vi "Create Custom Device.vi"(8 "error in (no error)":errorcluster, 9 "J1939 Monitor Settings":T2 {"Name" format="%.0x"}, 10 "J1939 XNET Settings":T3={"Database"="", "Cluster"="", "Port"="", "Baud rate [Bd]"=0, "Termination"=0, "Incoming Rate"=0, "Outcoming Rate"=0, "Write Decimation"=100} {"Termination" items=["Off", "On"]}, 11 "Device Item Ref in":T1 format="%.0x") -> (0 "error out":errorcluster, 2 "Monitor Ref out":T1 format="%.0x", 3 "Device Item Ref out":T1 format="%.0x")   [LabVIEW 2015, in "J1939 System Definition API Support.lvlib"]
uses:
  J1939 System Definition API Support.lvlib
  Shared/Types/XNET Settings.ctl
  Shared/Types/Monitor Settings.ctl
  <vilib>/NI Veristand/Custom Device API/Custom Device Item Ref.ctl
  Shared/SubVIs/Constants.vi
  <vilib>/NI/NIVS System Definition Utilities/_SubVIs/SysDef.Property.Set.Variant.vi
  Shared/J1939 Addon Shared.lvlib
  <vilib>/NI/NIVS System Definition Utilities/System Definition Utilities.lvlib
  <vilib>/NI VeriStand/Custom Device API/Custom Device API.lvlib
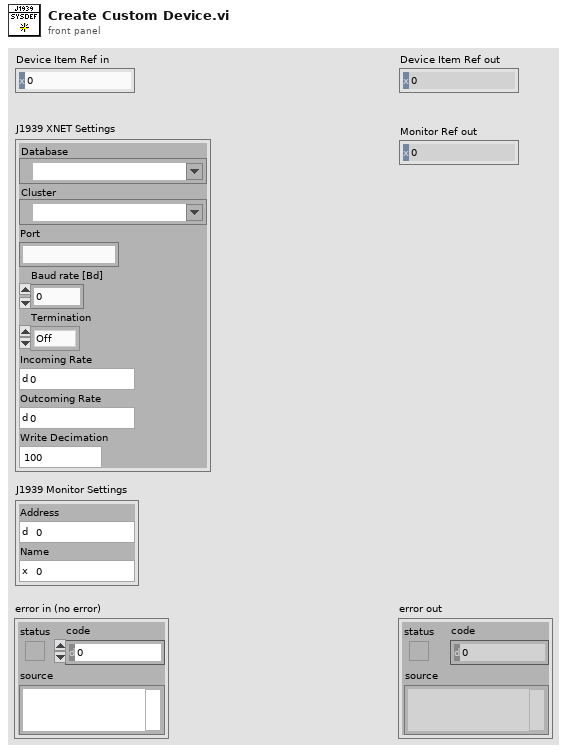
[diagram p1: front panel]
types:
  T1 = typedef "Custom Device API.lvlib/Custom Device Item Ref.ctl" = u64
  T2 = typedef "J1939 Addon Shared.lvlib/Monitor Settings.ctl" = cluster{"Address":u8, "Name":u64}
  T3 = typedef "J1939 Addon Shared.lvlib/XNET Settings.ctl" = cluster{"Database":refnum<k21>, "Cluster":refnum<k21>, "Port":string, "Baud rate [Bd]":u32, "Termination":u32, "Incoming Rate":u32, "Outcoming Rate":u32, "Write Decimation":u32}
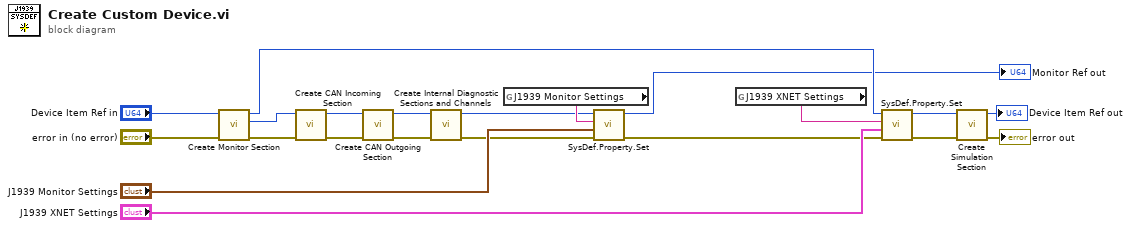
[diagram p0: block diagram]
diagram:
  n1 = call "Create Monitor Section.vi"("error in (no error)"="error in (no error)", "Device Item Ref in"="Device Item Ref in") -> ("error out"=w15:errorcluster, "Section Ptr"=w14:T1, "Parent Ref out"=w11:T1)  [unwired: 7 in]
  n2 = call "Create CAN Incoming Section.vi"("error in (no error)"=w15, "Device Item Ref in"=w14) -> ("error out"=w18:errorcluster, "Device Item Ref Out"=w19:T1)  [unwired: 8 in]
  n3 = call "Create CAN Outgoing Section.vi"("error in (no error)"=w18, "Parent Ref in"=w19) -> ("error out"=w21:errorcluster, "Parent Ref out"=w20:T1)  [unwired: 8 in]
  n4 = call "Create Internal Diagnostic Sections and Channels.vi"("error in (no error)"=w21, "Device Item Ref in"=w20) -> ("error out"=w7:errorcluster, "Device Item Ref Out"=w5:T1)  [unwired: 8 in]
  n5 = global read "Constants.vi" "J1939 Monitor Settings"() -> (w9:string)
  n6 = call-poly <vilib>:"SysDef.Property.Set.vi"("error in (no error)"=w7, "Value"="J1939 Monitor Settings", "Property Name"=w9, "nodeID"=w5) -> ("error out"=w6:errorcluster, "nodeID out"=→"Monitor Ref out":u64)  [unwired: 6 in]
  n7 = global read "Constants.vi" "J1939 XNET Settings"() -> (w17:string)
  n8 = call-poly <vilib>:"SysDef.Property.Set.vi"("error in (no error)"=w6, "Value"="J1939 XNET Settings", "Property Name"=w17, "nodeID"=w11) -> ("error out"=w13:errorcluster, "nodeID out"=w10:u64)  [unwired: 6 in]
  n9 = call "Create Simulation Section.vi"("error in (no error)"=w13, "Parent Ref in"=w10) -> ("error out"=→"error out":errorcluster, "Parent Ref out"=→"Device Item Ref out":T1)  [unwired: 7 in, 1 out]
